vi "Test Create table.vi"(8 "error in (no error)":errorcluster, 11 "TestCase in":refnum<class "Unit Testing.lvclass">) -> (0 "error out":errorcluster, 3 "TestCase out":refnum<class "Unit Testing.lvclass">)   [LabVIEW 2020, in "Unit Testing.lvclass"]
uses:
  Unit Testing.lvclass
  <vilib>/drjdpowell/SQLite Library/SQL Connection/Open (path).vi
  <vilib>/drjdpowell/SQLite Library/SQL Connection/Open (string).vi
  <vilib>/AdvancedString/Path To Command Line String.vi
  <vilib>/drjdpowell/SQLite Library/SQL Connection/Execute SQL (No results).vi
  <vilib>/drjdpowell/SQLite Library/SQL Connection/Connection.lvclass
  <vilib>/addons/_JKI Toolkits/VI Tester/TestCase.llb/TestCase.lvclass
  Contabilidad/Contabilidad.lvlib
  <vilib>/drjdpowell/SQLite Library/SQLite.lvlib
  C:/Program Files (x86)/National Instruments/LabVIEW 2020/vi.lib/addons/_JKI Toolkits/VI Tester/TestCase.llb/TestCase.lvclass
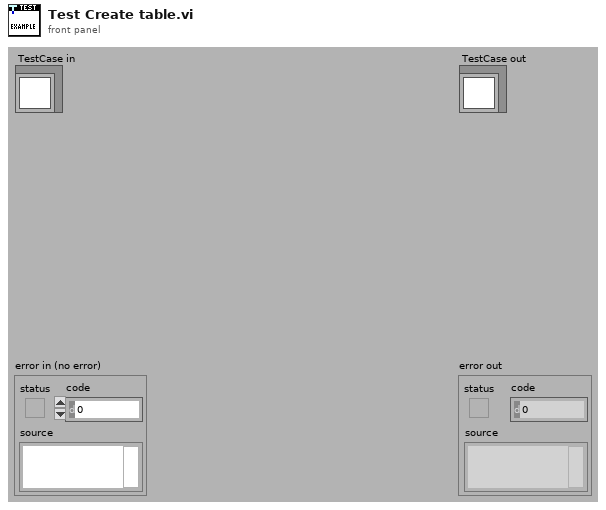
[diagram p1: front panel]
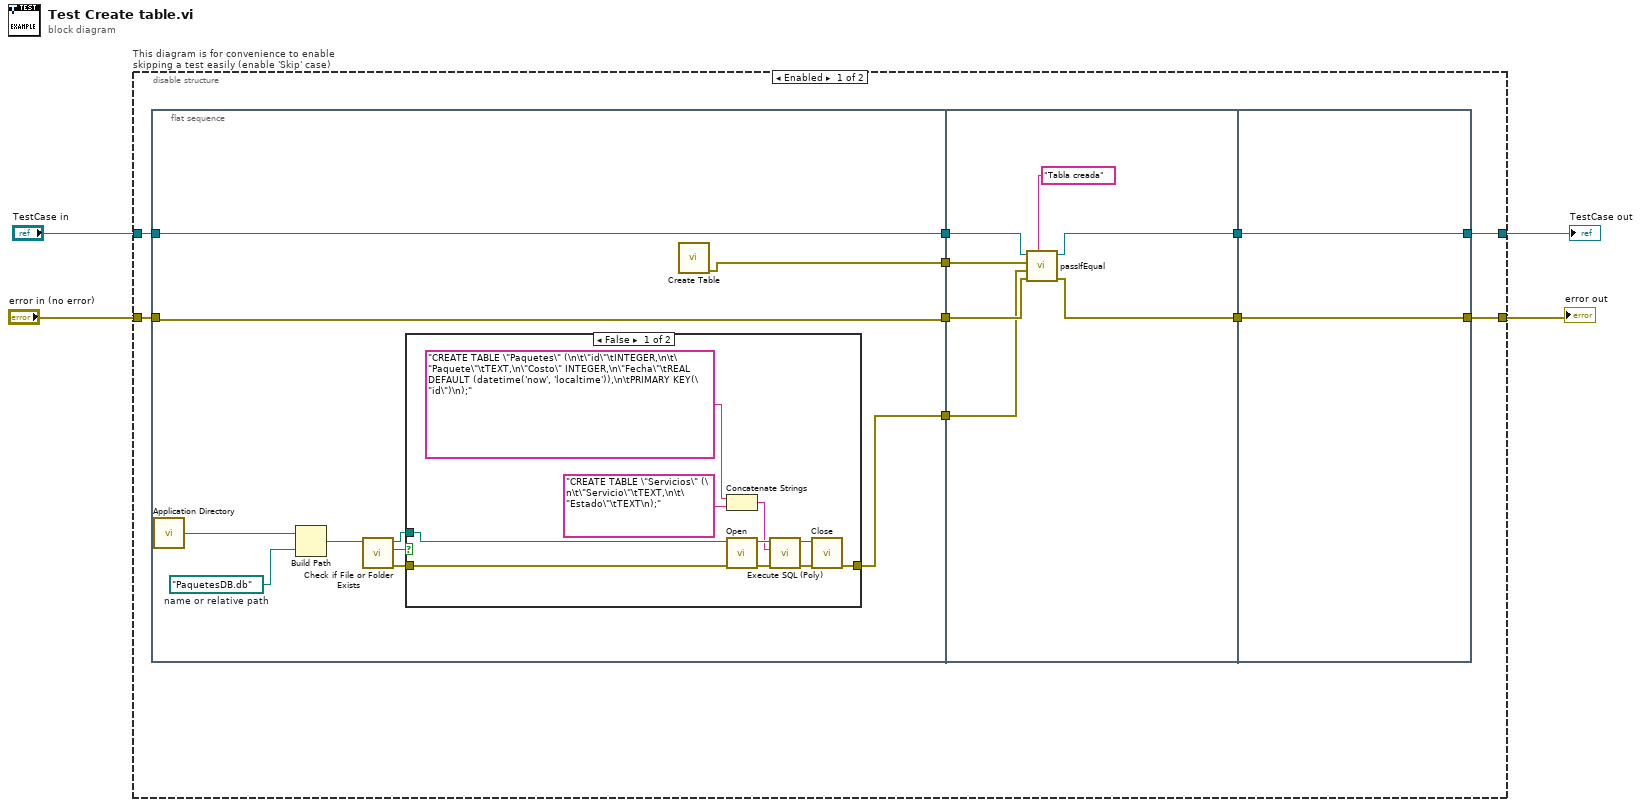
[diagram p0: block diagram]
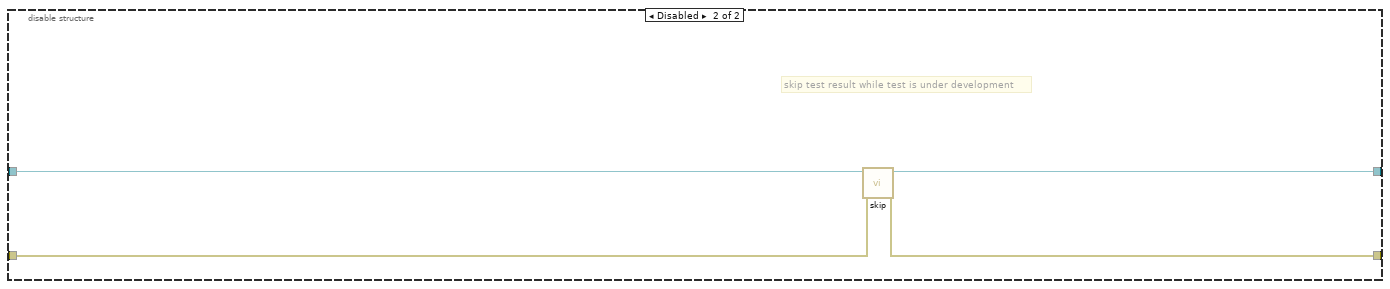
[diagram p3: hidden frame]
diagram:
  n1 = disable-structure "This diagram is for convenience to enable skipping a test easily (enable 'Skip' case)" shown="Enabled" {
    disable-tunnel: "TestCase in" -> [w8 w48]
    disable-tunnel: [w6 w46] -> w1
    disable-tunnel: [w5 w47] -> w3
    disable-tunnel: "error in (no error)" -> [w7 w45]
    frame Enabled {
      n2 = flat-sequence {
        tunnel: [w24] -> w14
        tunnel: w8 -> [w24]
        tunnel: [w23] -> w13
        tunnel: w7 -> [w23]
        tunnel: [w22] -> w12
        tunnel: [w15] -> w11
        tunnel: w14 -> [w42]
        tunnel: w13 -> [w41]
        tunnel: [w40] -> w10
        tunnel: [w39] -> w9
        tunnel: w12 -> [w37]
        tunnel: w11 -> [w38]
        tunnel: w10 -> [w44]
        tunnel: [w44] -> w5
        tunnel: [w43] -> w6
        tunnel: w9 -> [w43]
        frame #0 {
          w16 = path "PaquetesDB.db"  # name or relative path
          n3 = call <vilib>:"Application Directory.vi"() -> ("Application Directory"=w18:path)
          n4 = Build Path(base path=w18, name or relative path=w16) -> (appended path=w17:path)
          n5 = call <vilib>:"Check if File or Folder Exists.vi"("path"=w17) -> ("error out"=w19:errorcluster, "file or folder exists?"=w20:bool, "dup path"=w21:path)  [unwired: 8 in]
          n6 = case shown="False" w20 {
            tunnel: [w30 w35] -> w15
            tunnel: w21 -> [w28 _]
            tunnel: w19 -> [w29 w35]
            frame False {
              n7 = Concatenate Strings("CREATE TABLE \"Paquetes\" (\n\t\"id\"\tINTEGER,\n\t\"Paquete\"\tTEXT,\n\"Costo\" INTEGER,\n\"Fecha\"\tREAL DEFAULT (datetime('now', 'localtime')),\n\tPRIMARY KEY(\"id\")\n);", "CREATE TABLE \"Servicios\" (\n\t\"Servicio\"\tTEXT,\n\t\"Estado\"\tTEXT\n);") -> (w25:string)
              n8 = call-poly <vilib>:"Open.vi"("error in (no error)"=w29, "db file"=w28) -> ("error out"=w34:errorcluster, "SQLite Connection"=w33:refnum<class "Connection.lvclass">)  [unwired: 8 in]
              n9 = call-poly <vilib>:"Execute SQL (Poly).vi"("error in (no error)"=w34, "SQL"=w25, "SQLite Connection in"=w33) -> ("error out"=w32:errorcluster, "SQLite Connection"=w31:refnum<class "Connection.lvclass">)  [unwired: 7 in]
              n10 = call-dynamic "Close.vi"("error in (no error)"=w32, "SQLite Connection in"=w31) -> ("error out"=w30:errorcluster)  [unwired: 9 in]
            }
            frame True {
            }
          }
          n11 = call "Create Table.vi"() -> ("error out"=w22:errorcluster)  [unwired: 11 in]
        }
        frame #1 {
          n12 = call-dynamic "passIfEqual.vi"("custom report message (\"\")"="Tabla creada" ("custom report message (\"\")"), "error in (no error)"=w41, "y"=w38, "x"=w37, "TestCase in"=w42) -> ("error out"=w40:errorcluster, "TestCase out"=w39:refnum<class "Unit Testing.lvclass">)  [unwired: 5 in]
        }
        frame #2 {
        }
      }
    }
    frame Disabled {
      # "skip test result while test is under development"
      n13 = call <vilib>:"skip.vi"("error in (no error)"=w45, "TestCase in"=w48) -> ("error out"=w47:errorcluster, "TestCase out"=w46:refnum<class "Unit Testing.lvclass">)  [unwired: 8 in]
    }
  }
  "error out" <- w3
  "TestCase out" <- w1
